vi "RMS (CDB).vi"(0 "X":cdb[](array[numeric])) -> (1 "rms value":dbl, 2 "error":i32)   [LabVIEW 2020, in "NI_AALPro.lvlib"]
doc: "Computes the root mean square (rms) of the input sequence <B>X</B>."
uses:
  <vilib>/Analysis/NI_AALPro.lvlib
  <resource>/lvanlys.dll
panel:
  # "Complex RMS"
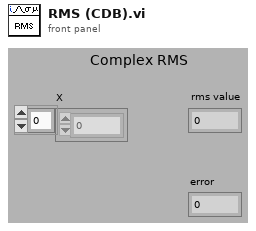
[diagram p1: front panel]
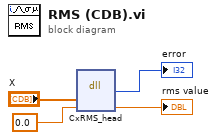
[diagram p0: block diagram]
diagram:
  n1 = dll-call lib="e:/builds/penguin/labview/branches/2020/dev/dist/resource/lvanlys.*" fn="CxRMS_head"("xH"="X", "rms"=0.0) -> ("return type"=→"error":i32, "rms"=→"rms value":dbl)  [unwired: 4 in, 2 out]
